vi "Overlay Dotted Line v1.vi"(0 "Imae in":T1, 1 "Color":u32(colorbox)=16711680, 5 "Line":T2 {"Start X" scale=0.0..1024.0; "End X" scale=0.0..1024.0}, 7 "Measurement Name":string, 9 "alternative factor":i32=20, 11 "error in (no error)":errorcluster, 12 "Point Diameter (5)":u32=18) -> (4 "Image":T1(plugin-control), 15 "error out":errorcluster)   [LabVIEW 2019]
uses:
  <vilib>/vision/Image Controls.llb/IMAQ Image.ctl
  <vilib>/vision/NI_Vision_Development_Module.lvlib
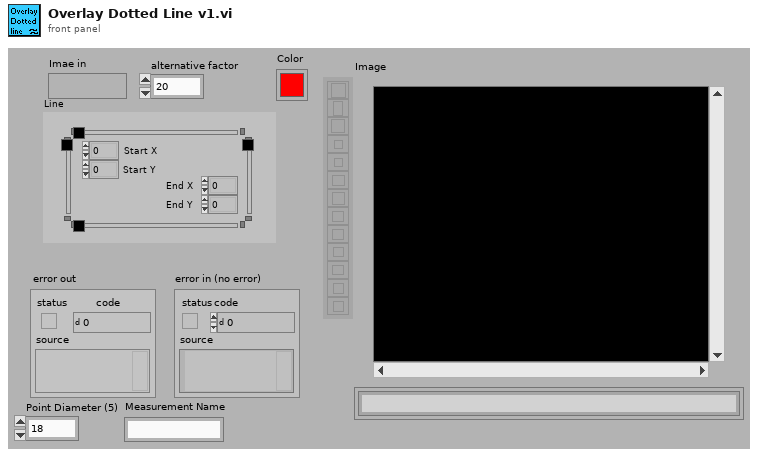
[diagram p1: front panel]
types:
  T1 = typedef "IMAQ Image.ctl" = refnum<image>
  T2 = typedef "IMAQ Line" = cluster{"Start X":i32, "Start Y":i32, "End X":i32, "End Y":i32}
  T3 = typedef "ROI Descriptor" = cluster{"Global Rectangle":i32[], "Contours":cluster{"ID":enum32{"External", "Internal"}, "Type":u32, "Coordinates":i32[]}[]}
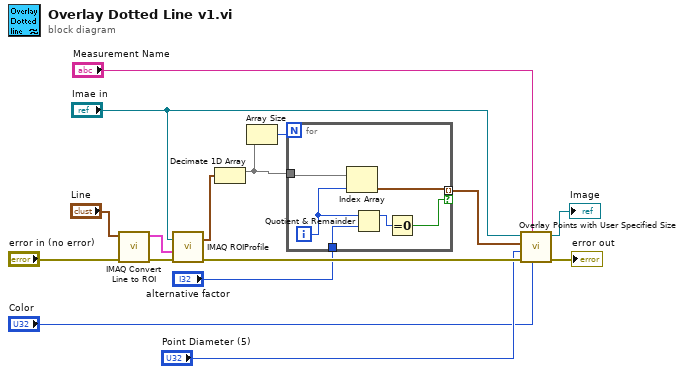
[diagram p0: block diagram]
diagram:
  n1 = call "IMAQ Convert Line to ROI"("error in (no error)"="error in (no error)", "Line"="Line") -> ("error out"=w14:errorcluster, "ROI Descriptor"=w15:T3)  [unwired: 7 in]
  n2 = call "IMAQ ROIProfile"("error in (no error)"=w14, "ROI Descriptor"=w15, "Image"="Imae in") -> ("error out"=w12:errorcluster, "Pixel Coordinates"=w5:cluster{"X":u32, "Y":u32}[])  [unwired: 1 in, 3 out]
  n3 = Decimate 1D Array(w5) -> (w3:cluster{"X":u32, "Y":u32}[])  [unwired: 1 out]
  n4 = Array Size(array=w3) -> (size(s)=w6:i32)
  n5 = for {
    N: w6 -> [_]
    tunnel: w3 -> [w22]
    tunnel: [w21] -> w7 mode=indexing if=w19
    tunnel: "alternative factor" -> [w20]
    i -> [w17]
    n6 = Index Array(array=w22, index=w17) -> (element=w21:cluster{"X":u32, "Y":u32})
    n7 = Quotient & Remainder(x=w17, y=w20) -> (x-y*floor(x/y)=w18:i32)  [unwired: 1 out]
    n8 = Equal To 0?(x=w18) -> (x = 0?=w19:bool)
  }
  n9 = call "Overlay Points with User Specified Size.vi"("Color"="Color", "Group"="Measurement Name", "error in"=w12, "Point Diameter (5)"="Point Diameter (5)", "Points"=w7, "Image In"="Imae in") -> ("error out"=→"error out":errorcluster, "Image Out"=→"Image":T1)  [unwired: 4 in]
